vi "Stop_set.vi"(8 "error in (no error)":errorcluster, 10 "Stop? (F)":bool) -> (0 "error out":errorcluster)   [LabVIEW 2009, in "NetworkVarTarget.lvlib"]
uses:
  NetworkVarTarget.lvlib
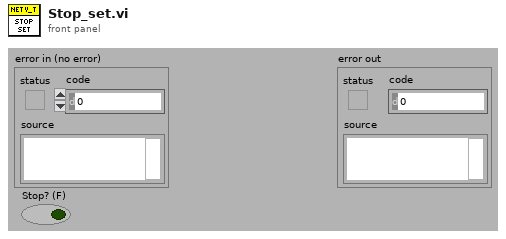
[diagram p1: front panel]
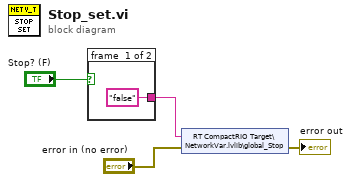
[diagram p0: block diagram]
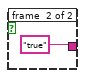
[diagram p2: hidden frame]
diagram:
  n1 = case shown="False" "Stop? (F)" {
    tunnel: ["false" ("global_Stop") "true" ("global_Stop")] -> w1
    frame #0 {
    }
    frame #1 {
    }
  }
  n2 = shared-variable "RT CompactRIO Target\\NetworkVar.lvlib\\global_Stop"(w1, error in="error in (no error)") -> (error out=→"error out":errorcluster)
